vi "Write Key.vi"(8 "error in (no error)":errorcluster, 10 "Key":u8(ring), 11 "Keyboard Action in":refnum<class "Keyboard Action.lvclass">) -> (0 "error out":errorcluster, 3 "Keyboard Action out":refnum<class "Keyboard Action.lvclass">)   [LabVIEW 2020, in "MacroAssert.lvlib" / "Keyboard Action.lvclass"]
uses:
  Keyboard Action.lvclass
  Keyboard Action.lvclass/Keyboard Action.ctl
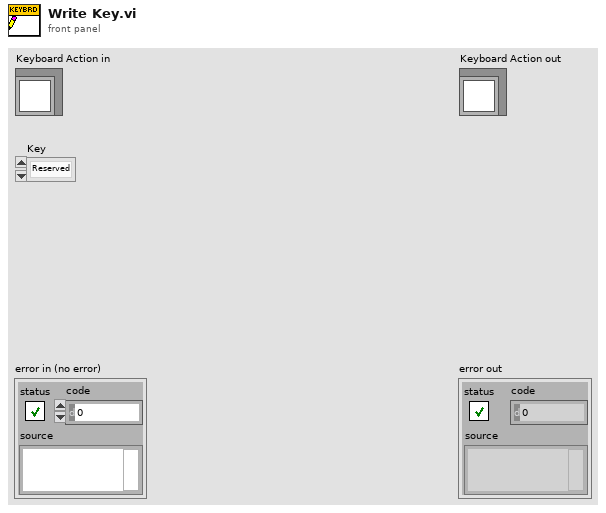
[diagram p1: front panel]
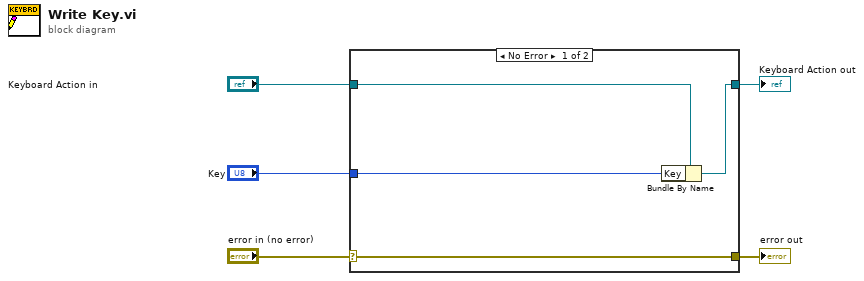
[diagram p0: block diagram]
diagram:
  n1 = case shown="No Error" "error in (no error)" {
    selector: "error in (no error)" -> [w9 w10]
    tunnel: [w9 w10] -> w4
    tunnel: [w7 w11] -> w2
    tunnel: "Keyboard Action in" -> [w8 w11]
    tunnel: "Key" -> [w6 _]
    frame No Error {
      n2 = Bundle By Name(cluster=w8, "Key"=w6) -> (w7:refnum<class "Keyboard Action.lvclass">)
    }
    frame Error {
    }
  }
  "error out" <- w4
  "Keyboard Action out" <- w2
